vi "ProcessDataFlow.vi"(7 "Qbus in":refnum<class "Qbus.lvclass">, 8 "error in (no error)":errorcluster, 10 "Data":T5, 11 "config in":T1={"Common"={"State"=enum."On", "Waveform Channel"="", "DataGroup"="", "Number of Samples"=0, "Waveform Length (sec)"=0.0, "Timeout"=0.0, "History"=variant, "LastRequest"=timestamp(0 s since 1904-01-01), "BufferSize"=0, "OpState"=variant, "IRoutingSource"={"CorrelationId"="", "ReplyTo"=""}}, "ChanNameMap"=variant}) -> (0 "error out":errorcluster, 3 "config out":T1={"Common"={"State"=enum."On", "Waveform Channel"="", "DataGroup"="", "Number of Samples"=0, "Waveform Length (sec)"=0.0, "Timeout"=0.0, "History"=variant, "LastRequest"=timestamp(0 s since 1904-01-01), "BufferSize"=0, "OpState"=variant, "IRoutingSource"={"CorrelationId"="", "ReplyTo"=""}}, "ChanNameMap"=variant})   [LabVIEW 2017, in "CmsTestPanel.lvlib"]
uses:
  <vilib>/addons/InsightCM/Devices/Shared/Cms/CmsTestPanel/CmsTestPanel.lvlib
  <vilib>/addons/InsightCM/Devices/Shared/Cms/CmsTestPanel/controls/Configuration.ctl
  <vilib>/addons/InsightCM/Devices/Shared/Common/TestPanel/controls/Configuration.ctl
  <vilib>/addons/InsightCM/Devices/Shared/Common/TestPanel/controls/State.ctl
  <vilib>/addons/InsightCM/MessageBus/Base/controls/IRoutingSource.ctl
  <vilib>/addons/InsightCM/Devices/Shared/Common/DataFlow/controls/Data.ctl
  <vilib>/addons/InsightCM/Utilities/DataAccessors/controls/wfmSGL_DVR.ctl
  <vilib>/addons/PointValueMap/controls/PointMap.ctl
  <vilib>/addons/InsightCM/Devices/Shared/Common/DataFlow/controls/Type.ctl
  <vilib>/addons/Qbus/Qbus.lvclass
  <vilib>/addons/InsightCM/MessageBus/MessageLibrary/Device/controls/DeviceTestPanelGetDataSetForChannelResponseBody.ctl
  <vilib>/addons/InsightCM/MessageBus/Base/controls/DataSetByteData.ctl
  <vilib>/addons/InsightCM/MessageBus/Base/controls/KeyValuePair.ctl
  <vilib>/addons/InsightCM/Devices/Shared/Common/ServerComm/ServerComm.lvlib
  <vilib>/addons/InsightCM/Devices/Shared/Common/TestPanel/TestPanel.lvlib
  <vilib>/addons/InsightCM/Devices/Shared/Common/DataFlow/DataFlow.lvlib
  <vilib>/addons/PointValueMap/PointValueMap.lvlib
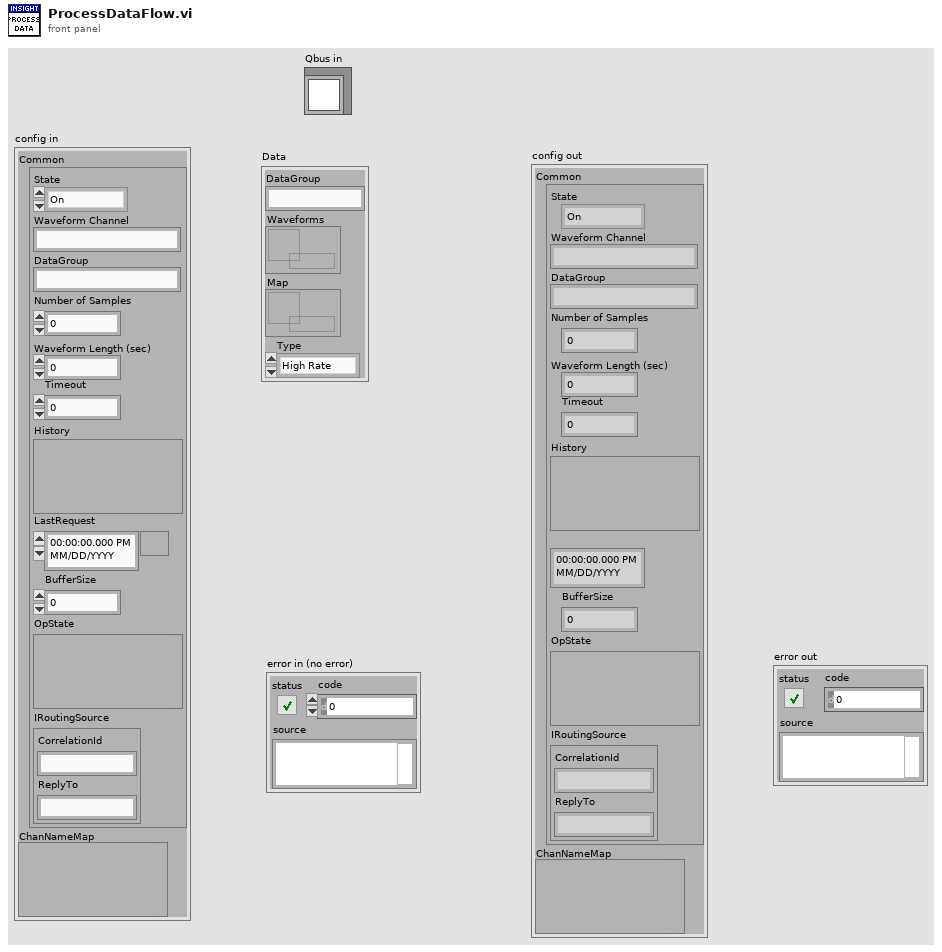
[diagram p1: front panel]
types:
  T1 = typedef "CmsTestPanel.lvlib/Configuration.ctl" = cluster{"Common":T2, "ChanNameMap":variant}
  T2 = typedef "TestPanel.lvlib/Configuration.ctl" = cluster{"State":T3, "Waveform Channel":string, "DataGroup":string, "Number of Samples":i32, "Waveform Length (sec)":dbl, "Timeout":dbl, "History":variant, "LastRequest":timestamp, "BufferSize":i32, "OpState":variant, "IRoutingSource":T4}
  T3 = typedef "TestPanel.lvlib/State.ctl" = enum16{"Off", "On", "PendingValues", "PendingDataSet"}
  T4 = typedef "IRoutingSource.ctl" = cluster{"CorrelationId":string, "ReplyTo":string}
  T5 = typedef "DataFlow.lvlib/Data.ctl" = cluster{"DataGroup":string, "Waveforms":T6, "Map":T7, "Type":T8}
  T6 = typedef "wfmSGL_DVR.ctl" = refnum<data-value>
  T7 = typedef "PointValueMap.lvlib/PointMap.ctl" = refnum<data-value>
  T8 = typedef "DataFlow.lvlib/Type.ctl" = enum16{"High Rate", "Low Rate", "Burst Mode"}
  T9 = typedef "DeviceTestPanelGetDataSetForChannelResponseBody.ctl" = cluster{"DataSet":T10}
  T10 = typedef "DataSetByteData.ctl" = cluster{"Id":string, "DataEventId":string, "AssetNodeId":string, "Type":string, "T0":i64, "Props":T11[], "DataBase64":string}
  T11 = typedef "KeyValuePair.ctl" = cluster{"Key":string, "Value":string}
  T12 = typedef "Message.ctl" = cluster{"Header":T13, "Body":u8[]}
  T13 = typedef "MessageHeader.ctl" = cluster{"MessageName":string, "Timestamp":i64, "CorrelationId":string, "ContentType":string, "RoutingKey":string, "Properties":T11[]}
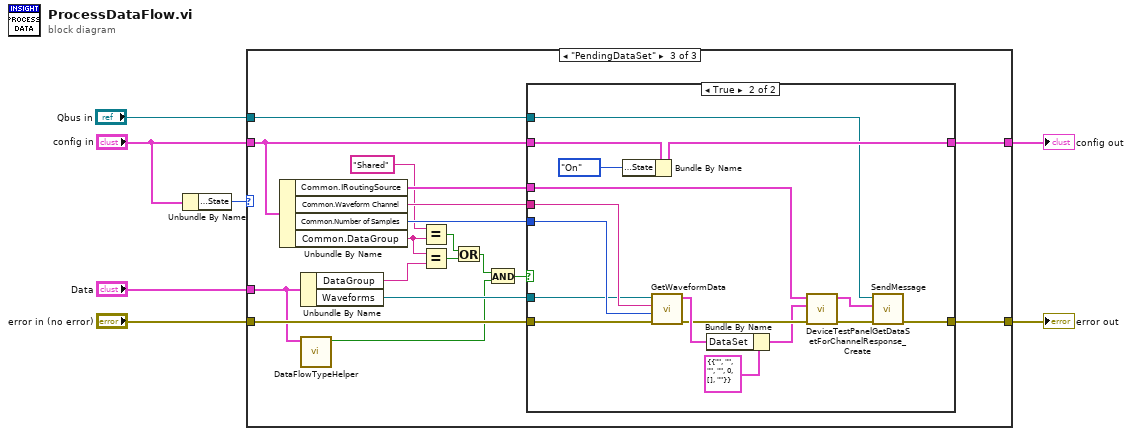
[diagram p0: block diagram]
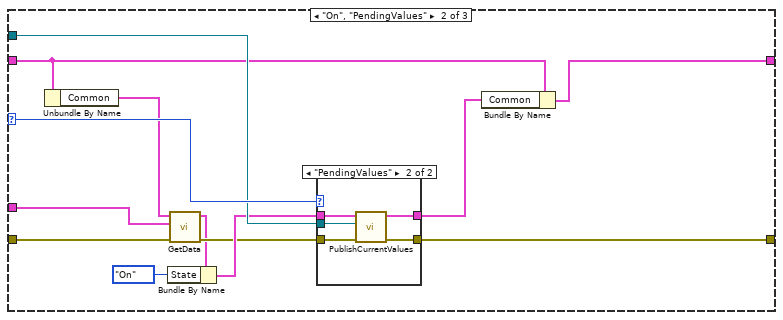
[diagram p3: hidden frame]
diagram:
  n1 = Unbundle By Name("config in") -> ("Common.State"=w7:T3)
  n2 = case shown="\"PendingDataSet\"" w7 {
    selector: w7 -> [_ w22 _]
    tunnel: "error in (no error)" -> [w8 w18 w47]
    tunnel: [w8 w21 w40] -> w2
    tunnel: "config in" -> [w9 w12 w43]
    tunnel: "Data" -> [_ w17 w31]
    tunnel: [w9 w10 w42] -> w3
    tunnel: "Qbus in" -> [_ w20 w41]
    frame "Off" {
    }
    frame "On", "PendingValues" {
      n3 = Unbundle By Name(w12) -> ("Common"=w16:T2)
      n4 = call <vilib>:"GetData.vi"("error in (no error)"=w18, "Data"=w17, "config in"=w16) -> ("error out"=w15:errorcluster, "config out"=w14:T2)  [unwired: 7 in]
      n5 = Bundle By Name(cluster=w14, "State"=State."On" ("Test Panel State")) -> (w19:T2)
      n6 = case shown="\"PendingValues\"" w22 {
        tunnel: w19 -> [w23 w27]
        tunnel: w15 -> [w24 w29]
        tunnel: [w24 w28] -> w21
        tunnel: [w23 w25] -> w11
        tunnel: w20 -> [_ w26]
        frame Default {
        }
        frame "PendingValues" {
          n7 = call <vilib>:"PublishCurrentValues.vi"("error in (no error)"=w29, "Qbus in"=w26, "config in"=w27) -> ("error out"=w28:errorcluster, "config out"=w25:T2)  [unwired: 7 in]
        }
      }
      n8 = Bundle By Name(cluster=w12, "Common"=w11) -> (w10:T1)
    }
    frame "PendingDataSet" {
      n9 = Unbundle By Name(w43) -> ("Common.IRoutingSource"=w39:T4, "Common.Waveform Channel"=w46:string, "Common.Number of Samples"=w45:i32, "Common.DataGroup"=w36:string)
      n10 = Unbundle By Name(w31) -> ("DataGroup"=w38:string, "Waveforms"=w44:T6)
      n11 = call <vilib>:"DataFlowTypeHelper.vi"("data"=w31) -> ("high rate"=w30:bool)  [unwired: 8 in, 2 out]
      n12 = Equal?(x="Shared", y=w36) -> (x = y?=w35:bool)
      n13 = Equal?(x=w36, y=w38) -> (x = y?=w37:bool)
      n14 = Or(x=w35, y=w37) -> (x .or. y?=w33:bool)
      n15 = And(x=w33, y=w30) -> (x .and. y?=w32:bool)
      n16 = case shown="True" w32 {
        tunnel: w47 -> [w49 w65]
        tunnel: w46 -> [_ w64]
        tunnel: w45 -> [_ w63]
        tunnel: w44 -> [_ w62]
        tunnel: w43 -> [w48 w61]
        tunnel: [w48 w60] -> w42
        tunnel: w41 -> [_ w59]
        tunnel: [w49 w54] -> w40
        tunnel: w39 -> [_ w52]
        frame False {
        }
        frame True {
          n17 = Bundle By Name(cluster=w61, "Common.State"=State."On" ("Test Panel State")) -> (w60:T1)
          n18 = call <vilib>:"GetWaveformData.vi"("error in (no error)"=w65, "Number of Samples"=w63, "Current Channel"=w64, "Data Value Reference in"=w62) -> ("error out"=w55:errorcluster, "DataSet"=w57:T10)  [unwired: 6 in]
          n19 = Bundle By Name(cluster=T9 {"DataSet"={"Id"="", "DataEventId"="", "AssetNodeId"="", "Type"="", "T0"=0, "Props"=[], "DataBase64"=""}} ("DeviceTestPanelGetWaveformChannelResponse"), "DataSet"=w57) -> (w53:T9)
          n20 = call <vilib>:"DeviceTestPanelGetDataSetForChannelResponse_Create.vi"("error in (no error)"=w55, "DeviceTestPanelGetDataSetForChannelResponse"=w53, "IRoutingSource"=w52) -> ("error out"=w56:errorcluster, "Message"=w51:T12)  [unwired: 7 in]
          n21 = call <vilib>:"SendMessage.vi"("error in (no error)"=w56, "message"=w51, "Qbus in"=w59) -> ("error out"=w54:errorcluster)  [unwired: 7 in, 1 out]
        }
      }
    }
  }
  "error out" <- w2
  "config out" <- w3
